vi "Store Training and Testing set.vi"() -> ()   [LabVIEW 2020]
panel:
  in  "Store Training/testing set":bool
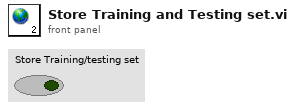
[diagram p1: front panel]
diagram:
